vi "FT-IR Scans SysLog.vi"(11 "(90) ftirScans":T1 format="%#_5g") -> (3 "(90) ftirScans out":T1 format="%#_5g")   [LabVIEW 2015, in "FT-IR.lvlib"]
uses:
  FT-IR.lvlib
  Visualisierungs Elemente/Zahlen-Eingabefeld.ctl
  FGV FT-IR Aktionen.ctl
  SysLog/SysLog Interface.ctl
  SysLog/SysLog.lvlib
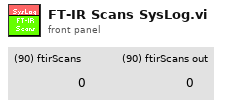
[diagram p1: front panel]
types:
  T1 = typedef "Zahlen-Eingabefeld.ctl" = sgl
  T2 = typedef "FT-IR.lvlib/FGV FT-IR Aktionen.ctl" = enum16{"lesen", "NOG setzen", "NOS setzen", "Initialisieren", "speichern", "ALLES setzen", "FT-IR Spektrum loggen", "Komm Stoppen"}
  T3 = typedef "SysLog.lvlib/SysLog Interface.ctl" = cluster{"FehlermeldungsCode":i32, "ErfolgsmeldungsCode":i32, "ParameterListenString":string, "Anzeige":bool, "SysLogIcon":enum16{"OK", "Warnung", "Fehler"}, "intern":bool}
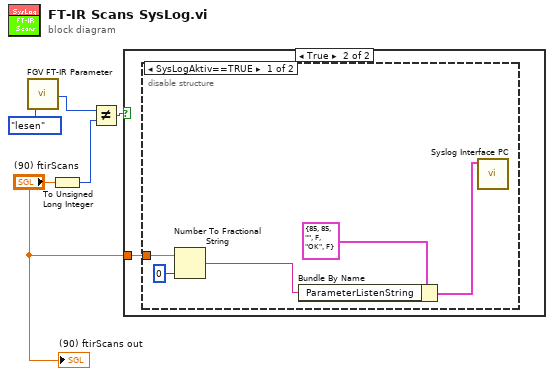
[diagram p0: block diagram]
diagram:
  n1 = call "FGV FT-IR Parameter.vi"("Aktion"=FGV_FT-IR_Aktionen."lesen") -> ("NoOfScan"=w4:u32)  [unwired: 11 in, 7 out]
  n2 = To Unsigned Long Integer(number="(90) ftirScans") -> (unsigned 32bit integer=w1:u32)
  n3 = Not Equal?(x=w4, y=w1) -> (x != y?=w2:bool)
  n4 = case shown="True" w2 {
    tunnel: "(90) ftirScans" -> [_ w6]
    frame False {
    }
    frame True {
      n5 = disable-structure shown="SysLogAktiv==TRUE" {
        disable-tunnel: w6 -> [w10 _]
        frame condition #0 (active) {
          n6 = Number To Fractional String(number=w10, precision (6)=i16 0 ("Genauigkeit (6)")) -> (F-format string=w8:string)  [unwired: 2 in]
          n7 = Bundle By Name(cluster=T3 {"FehlermeldungsCode"=85, "ErfolgsmeldungsCode"=85, "ParameterListenString"="", "Anzeige"=FALSE, "SysLogIcon"=enum."OK", "intern"=FALSE} ("Cluster (in)"), "ParameterListenString"=w8) -> (w7:T3)
          n8 = call "Syslog Interface PC.vi"("Cluster (in)"=w7) -> ()  [unwired: 10 in, 1 out]
        }
        frame condition #1 {
        }
      }
    }
  }
  "(90) ftirScans out" <- "(90) ftirScans"
